vi "test_save.vi"() -> ()   [LabVIEW 2016]
panel:
  in  "Boolean":bool
  out "String":string
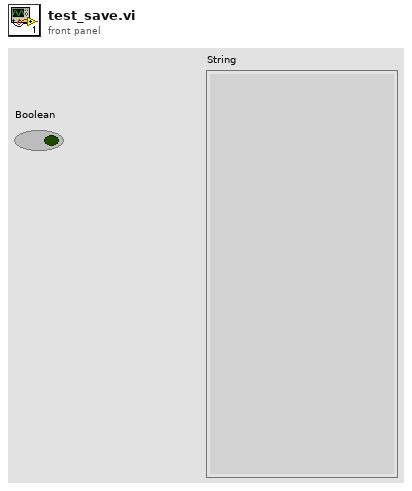
[diagram p1: front panel]
types:
  T1 = enum16{"open", "replace", "create", "open or create", "replace or create", "replace or create with confirmation"}
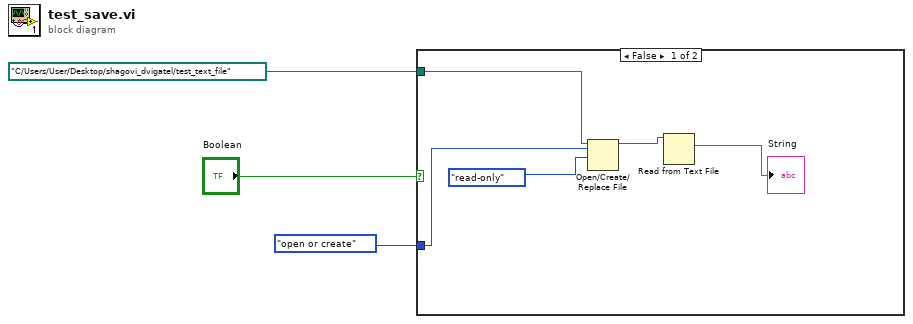
[diagram p0: block diagram]
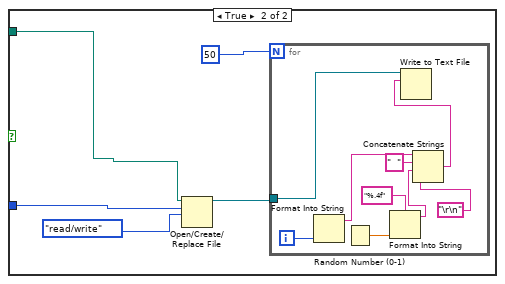
[diagram p2: hidden frame]
diagram:
  n1 = case shown="False" "Boolean" {
    tunnel: T1."open or create" ("operation (0:open)") -> [w6 w11]
    tunnel: path "C:/Users/User/Desktop/shagovi_dvigatel/test_text_file" -> [w4 w10]
    frame False {
      n2 = Open/Create/Replace File(file path (use dialog)=w4, operation (0:open)=w6, access (0:read/write)=enum16{"read/write", "read-only", "write-only"}."read-only") -> (refnum out=w8:refnum<file>)  [unwired: 3 in, 2 out]
      n3 = Read from Text File(file (use dialog)=w8) -> (text=→"String":string)  [unwired: 3 in, 3 out]
    }
    frame True {
      n4 = Open/Create/Replace File(file path (use dialog)=w10, operation (0:open)=w11, access (0:read/write)=enum16{"read/write", "read-only", "write-only"}."read/write") -> (refnum out=w13:refnum<file>)  [unwired: 3 in, 2 out]
      n5 = for {
        N: 50 -> [_]
        tunnel: w13 -> [w22]
        i -> [w20]
        n6 = Format Into String(w20) -> (resulting string=w19:string)  [unwired: 3 in, 1 out]
        n7 = Random Number (0-1)() -> (number: 0 to 1=w21:dbl)
        n8 = Format Into String(format string="%.4f", w21) -> (resulting string=w17:string)  [unwired: 2 in, 1 out]
        n9 = Concatenate Strings(w19, "  " ("string"), w17, "\r\n") -> (w15:string)
        n10 = Write to Text File(file (use dialog)=w22, text=w15) -> ()  [unwired: 2 in, 3 out]
      }
    }
  }
